vi "SRingThreadIsOFF_SD.vi"() -> (0 "ThreadIsOFF":u8)   [LabVIEW 2015]
uses:
  DLL/ESLSCDLL.dll
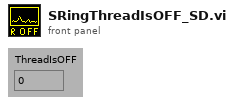
[diagram p1: front panel]
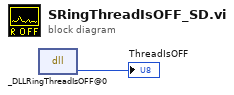
[diagram p0: block diagram]
diagram:
  n1 = dll-call lib="G:/SD/TRANCON-2015/DLL/ESLSCDLL.dll" fn="_DLLRingThreadIsOFF@0" ("lwlscdll.dll:DLLRingThreadIsOFF")() -> ("Rückgabetyp"=→"ThreadIsOFF":u8)  [unwired: 3 in, 2 out]
